vi "Add Observer.vi"(8 "error in (no error)":errorcluster, 11 "Observable Actor in":refnum<class "Observable Actor.lvclass">) -> (0 "error out":errorcluster, 2 "new observer":T1, 3 "Observable Actor out":refnum<class "Observable Actor.lvclass">)   [LabVIEW 2014, in "Observable Actor.lvlib" / "Observable Actor.lvclass"]
uses:
  Observable Actor.lvclass
  Observer.ctl
  Observable Actor.lvclass/Observable Actor.ctl
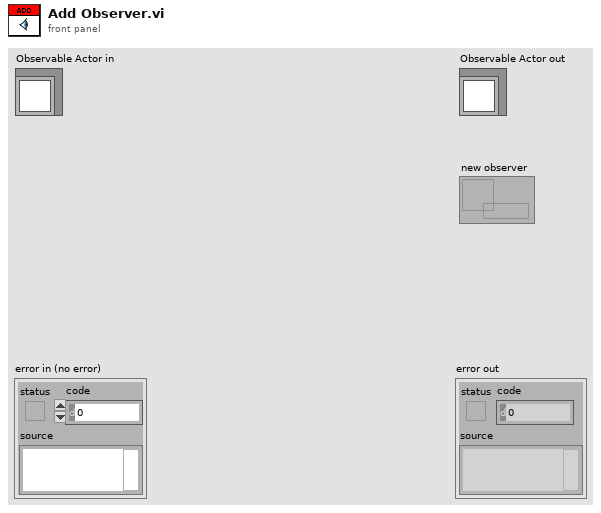
[diagram p1: front panel]
types:
  T1 = typedef "Observable Actor.lvlib/Observable Actor.lvclass/Observer.ctl" = refnum<queue>
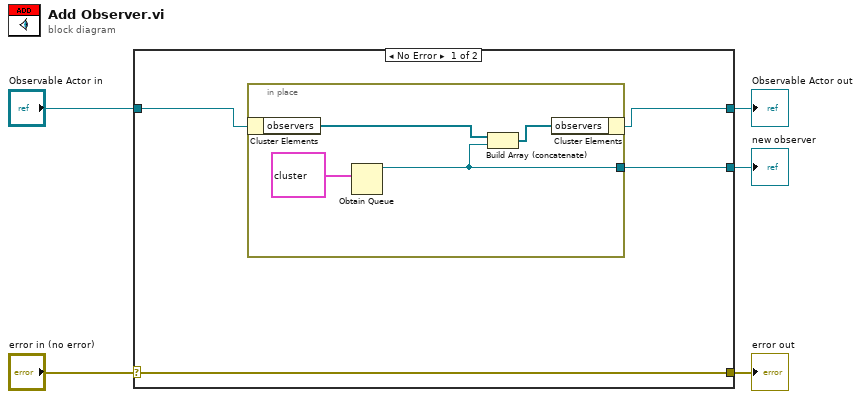
[diagram p0: block diagram]
diagram:
  n1 = case shown="No Error" "error in (no error)" {
    selector: "error in (no error)" -> [w9 w15]
    tunnel: [w9 w15] -> w4
    tunnel: [w7 w14] -> w2
    tunnel: "Observable Actor in" -> [w8 w14]
    tunnel: [w6 _] -> w1
    frame No Error {
      n2 = in-place {
        in-place-border: [w10] -> w6
        n3 = in-place-cluster #1(w8) -> ("observers"=w13:T1[])
        n4 = Obtain Queue(element data type=cluster{"value":variant, "name":string} {"value"=variant, "name"=""} ("output cluster")) -> (queue out=w10:refnum<queue>)  [unwired: 4 in, 2 out]
        n5 = Build Array (concatenate)(w13, w10) -> (w12:T1[])
        n6 = in-place-cluster #1("observers"=w12) -> (w7:refnum<class "Observable Actor.lvclass">)
      }
    }
    frame Error {
    }
  }
  "error out" <- w4
  "Observable Actor out" <- w2
  "new observer" <- w1
